vi "Testmec.vi"() -> ()   [LabVIEW 2013]
uses:
  <vilib>/Rock Robotics/SystemInterfaces/DIO/FPGA_DIOPWMChannel.ctl
  <vilib>/Rock Robotics/WPI/MotorControl/WPI_MotorControlOpen Talon.vi
panel:
  out "Output 2":dbl
  out "Output":dbl
  in  "stop":bool
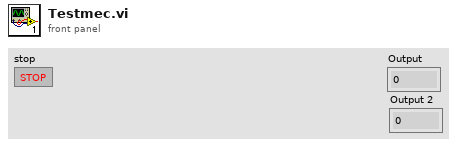
[diagram p1: front panel]
types:
  T1 = typedef "FPGA_DIOPWMChannel.ctl" = enum8{"PWM 1", "PWM 2", "PWM 3", "PWM 4", "PWM 5", "PWM 6", "PWM 7", "PWM 8", "PWM 9", "PWM 10", "Invalid"}
  T2 = typedef "WPI_MotorControlDeviceRef.ctl" = cluster{"DeviceStatus":errorcluster, "Type":enum16{"PWM", "CAN"}, "PWM":cluster{"Digital Module":T3, "PWM Channel":T1, "DeadBand":T4}, "CAN":cluster{"Device Number":u8, "Control Mode":T5, "Semaphore":T6, "Max Vout":dbl}, "Invert":bool, "TransformRef":T7, "InvTransformRef":T7}
  T3 = typedef "FPGA_TypedefDigitalModule.ctl" = enum16{"Digital Module 1", "Digital Module 2"}
  T4 = typedef "WPI_PWMDeadband.ctl" = cluster{"Name":string, "maxPositivePwm":i32, "minPositivePwm":i32, "centerPwm":i32, "maxNegativePwm":i32, "minNegativePwm":i32, "angularRange":u16}
  T5 = typedef "WPI_CANJaguar_ControlMode.ctl" = enum8{"Percent VBus", "Current", "Speed", "Position", "Voltage"}
  T6 = typedef "Semaphore RefNum" = refnum<k1>
  T7 = typedef "WPI_PWMTransform_ConPane.ctl" = refnum<vi>
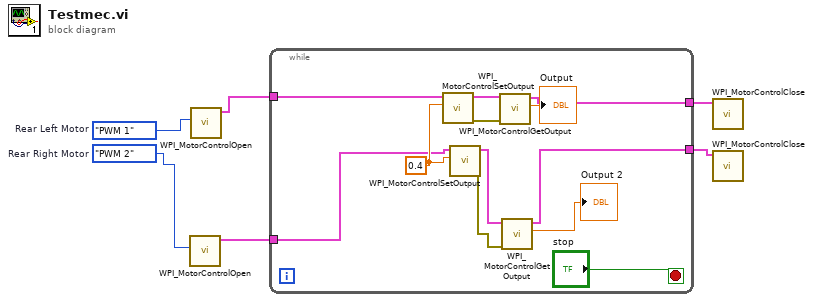
[diagram p0: block diagram]
diagram:
  w3 = FPGA_DIOPWMChannel."PWM 2"  # Rear Right Motor
  w4 = FPGA_DIOPWMChannel."PWM 1"  # Rear Left Motor
  n1 = call-poly <vilib>:"WPI_MotorControlOpen.vi"("PWM Channel"=w3) -> ("MotorControlDeviceRef"=w1:T2)  [unwired: 9 in, 1 out]
  n2 = call-poly <vilib>:"WPI_MotorControlOpen.vi"("PWM Channel"=w4) -> ("MotorControlDeviceRef"=w2:T2)  [unwired: 9 in, 1 out]
  n3 = while {
    tunnel: [w9] -> w6
    tunnel: [w12] -> w5
    tunnel: w2 -> [w16]
    tunnel: w1 -> [w15]
    stop <- "stop" stop-if-true
    w18 = 0.4 ("Output")
    n4 = call <vilib>:"WPI_MotorControlSetOutput.vi"("Output"=w18, "MotorControlDevRef"=w16) -> ("error out"=w11:errorcluster, "MotorControlDevRef"=w10:T2)  [unwired: 7 in, 1 out]
    n5 = call <vilib>:"WPI_MotorControlSetOutput.vi"("Output"=w18, "MotorControlDevRef"=w15) -> ("error out"=w14:errorcluster, "MotorControlDevRef"=w13:T2)  [unwired: 7 in, 1 out]
    n6 = call <vilib>:"WPI_MotorControlGetOutput.vi"("error in (no error)"=w11, "MotorControlDevRef"=w10) -> ("Output"=→"Output":dbl, "MotorControlDevRef"=w9:T2)  [unwired: 7 in, 1 out]
    n7 = call <vilib>:"WPI_MotorControlGetOutput.vi"("error in (no error)"=w14, "MotorControlDevRef"=w13) -> ("Output"=→"Output 2":dbl, "MotorControlDevRef"=w12:T2)  [unwired: 7 in, 1 out]
  }
  n8 = call <vilib>:"WPI_MotorControlClose.vi"("MotorControlDevRef"=w6) -> ()  [unwired: 10 in, 1 out]
  n9 = call <vilib>:"WPI_MotorControlClose.vi"("MotorControlDevRef"=w5) -> ()  [unwired: 10 in, 1 out]
